vi "Set Build Specification Description.vi"(8 "error in (no error)":errorcluster, 10 "Build Specification Description":string, 11 "NI_AB_API_Build in":refnum<class "NI_AB_API_Build.lvclass">) -> (0 "error out":errorcluster, 3 "NI_AB_API_Build out":refnum<class "NI_AB_API_Build.lvclass">)   [LabVIEW 2020, in "NI_AB_API_Build.lvclass"]
uses:
  <vilib>/AppBuilder/AB_API/Build/NI_AB_API_Build.lvclass
  <vilib>/AppBuilder/AB_API/Build/NI_AB_API_Build.lvclass/NI_AB_API_Build.ctl
  <vilib>/AppBuilder/AB_Classes/Build/AB_Build.lvclass
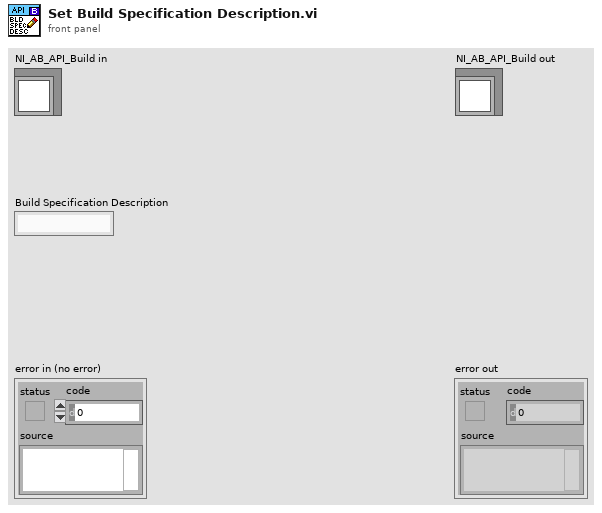
[diagram p1: front panel]
types:
  T1 = typedef "AB_Build.ctl" = cluster{"buildSpecName":string, "buildSpecDescription":string, "destinations":refnum<class "AB_Destination.lvclass">[], "exclusionOption":T2, "defaultLanguage":string, "supportedLanguages":string[], "excludedDirectories":path[], "buildContext":refnum<vi>, "buildObject":T3, "preview":bool, "programatic":bool, "progressBarEvents":T4, "userLog_Path":path, "preActionID":string, "preAction_Path":path, "postActionID":string, "postAction_Path":path, "eng_checkForBrokenVIs?":bool, "eng_verboseLinkerErrors?":bool, "localDest_Path":path, "targetDest_Path":path, "removeVIObject":u16, "cache":refnum<class "PreviewCache.lvclass">, "use cache":bool, "previewCache_ID":string, "buildCache_ID":string, "eng_TempLocalDest_Path":path, "eng_collectDependencies?":bool, "versionInfo":cluster{"buildVersion":cluster{"major":u16, "minor":u16, "patch":u16, "build":u16}, "autoIncrement":bool}, "eng_enableVIChecksums":bool}
  T2 = typedef "AB_Exclusion_Option.ctl" = cluster{"typedefs":bool, "polymorphicVIs":bool, "unusedLibraryItems":bool, "modifyLibraryFile":bool, "edit-timeDependencies":bool, "inlineVIs":bool, "dependent PPLs":bool, "dependent DLLs":bool}
  T3 = typedef "ItemRef.ctl" = u64
  T4 = typedef "provcom_ProgressBar_Events.ctl" = cluster{"newJob":refnum<user-event>, "newItem":refnum<user-event>, "errorMsg":T5, "cancel":refnum<user-event>}
  T5 = typedef "mxLvBuildError.ctl" = refnum<user-event>
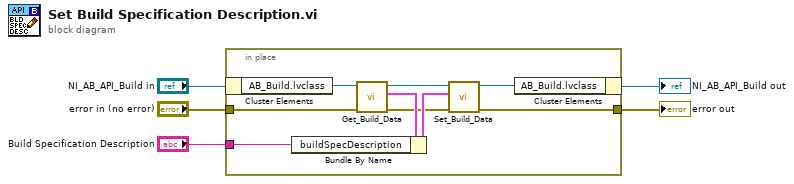
[diagram p0: block diagram]
diagram:
  n1 = in-place {
    in-place-border: [w14] -> w4
    in-place-border: "error in (no error)" -> [w13]
    in-place-border: "Build Specification Description" -> [w6]
    n2 = in-place-cluster #1("NI_AB_API_Build in") -> ("AB_Build.lvclass"=w7:refnum<class "AB_Build.lvclass">)
    n3 = call <vilib>:"Get_Build_Data.vi"("error in (no error)"=w13, "Class in"=w7) -> ("error out"=w9:errorcluster, "data"=w11:T1, "Class out"=w12:refnum<class "AB_Build.lvclass">)  [unwired: 7 out]
    n4 = Bundle By Name(cluster=w11, "buildSpecDescription"=w6) -> (w10:T1)
    n5 = call <vilib>:"Set_Build_Data.vi"("error in (no error)"=w9, "data"=w10, "Class in"=w12) -> ("error out"=w14:errorcluster, "Class out"=w8:refnum<class "AB_Build.lvclass">)  [unwired: 7 out]
    n6 = in-place-cluster #1("AB_Build.lvclass"=w8) -> (→"NI_AB_API_Build out":refnum<class "NI_AB_API_Build.lvclass">)
  }
  "error out" <- w4
